vi "open_relay.vi"(3 "错误输入（无错误）":errorcluster, 4 "写入缓冲区":string, 5 "VISA资源名称":refnum<visa-resource-name>) -> (0 "返回数":u32, 1 "错误输出":errorcluster, 2 "VISA资源名称输出":refnum<visa-resource-name>)   [LabVIEW 2020]
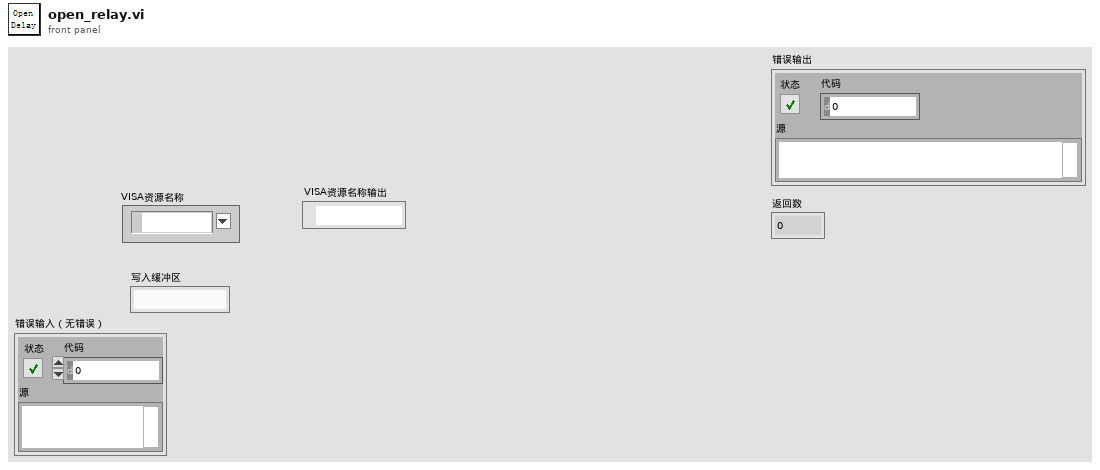
[diagram p1: front panel]
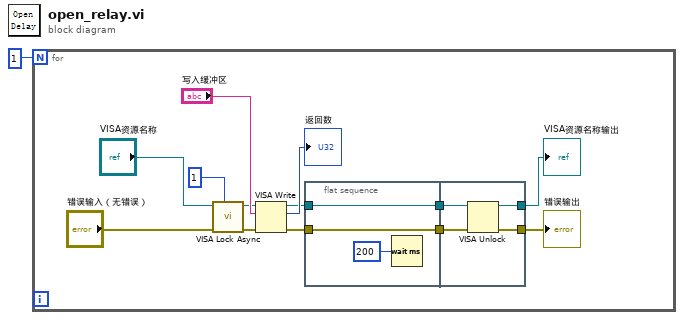
[diagram p0: block diagram]
diagram:
  n1 = for {
    N: 1 -> [_]
    n2 = call <vilib>:"VISA Lock Async.vi"("lock type (exclusive: 1)"=u32 1, "error in (no error)"="错误输入（无错误）", "VISA resource name"="VISA资源名称") -> ("error out"=w10:errorcluster, "VISA resource name out"=w12:refnum<visa-resource-name>)  [unwired: 6 in, 1 out]
    n3 = VISA Write(VISA resource name=w12, write buffer="写入缓冲区", error in (no error)=w10) -> (VISA resource name out=w2:refnum<visa-resource-name>, return count=→"返回数":u32, error out=w7:errorcluster)
    n4 = flat-sequence {
      tunnel: w7 -> [w17]
      tunnel: [w17] -> w4
      tunnel: [w15] -> w3
      tunnel: w2 -> [w15]
      tunnel: [w20] -> w6
      tunnel: [w19] -> w5
      tunnel: w4 -> [w21]
      tunnel: w3 -> [w18]
      frame #0 {
        n5 = Wait (ms)(milliseconds to wait=u32 200 ("等待时间（毫秒）")) -> ()  [unwired: 1 out]
      }
      frame #1 {
        n6 = VISA Unlock(8:w21, 11:w18) -> (0:w20:errorcluster, 3:w19:refnum<visa-resource-name>)
      }
    }
    "VISA资源名称输出" <- w5
    "错误输出" <- w6
  }
